vi "row to excel label.vi"() -> ()   [LabVIEW 2015]
uses:
  <vilib>/addons/_office/NI_ReportGenerationToolkit.lvlib
panel:
  out "cell's name":string
  in  "start (-1, -1) 2":cluster{"row":i32, "column":i32}={"row"=-1, "column"=-1}
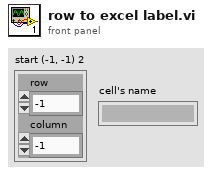
[diagram p1: front panel]
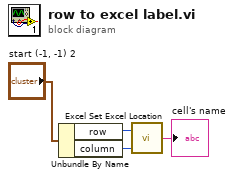
[diagram p0: block diagram]
diagram:
  n1 = Unbundle By Name("start (-1, -1) 2") -> ("row"=w3:i32, "column"=w2:i32)
  n2 = call <vilib>:"Excel Set Excel Location.vi"("column"=w2, "row"=w3) -> ("cell's name"=→"cell's name":string)
